vi "AllDataConcat.vi"(8 "error in (no error)":errorcluster, 11 "AllDataArray":T1[](array[typedef]) {"FlukeData"."DataAnalysisArray"."TimeStamp" format="%^<%.3X\n%x>T"; "FlukeData"."ModelDataArray"."FREQUENCY" format="%#_6f"; "FlukeData"."ModelDataArray"."TimeStamp" format="%^<%.3X\n%x>T"; "FlukeData"."PMUDataArray"."FREQUENCY" format="%#_6f"; "FlukeData"."PMUDataArray"."TimeStamp" format="%^<%.3X\n%x>T"; "NISTData"."DataAnlysisArray"."Time" format="%.6f"; "NISTData"."DataAnlysisArray"."TimeStamp" format="%^<%.3X\n%x>T"; "NISTData"."DUTDataArray"."TimeStamp" format="%^<%.3X\n%x>T"; "NISTData"."DUTDataArray"."Time" format="%.6f"; "NISTData"."NIDataArray"."TimeStamp" format="%^<%.3X\n%x>T"; "NISTData"."NIDataArray"."Time" format="%.6f"}) -> (0 "error out":errorcluster, 3 "AllData":T1 {"FlukeData"."DataAnalysisArray"."TimeStamp" format="%^<%.3X\n%x>T"; "FlukeData"."ModelDataArray"."FREQUENCY" format="%#_6f"; "FlukeData"."ModelDataArray"."TimeStamp" format="%^<%.3X\n%x>T"; "FlukeData"."PMUDataArray"."FREQUENCY" format="%#_6f"; "FlukeData"."PMUDataArray"."TimeStamp" format="%^<%.3X\n%x>T"; "NISTData"."DataAnlysisArray"."Time" format="%.6f"; "NISTData"."DataAnlysisArray"."TimeStamp" format="%^<%.3X\n%x>T"; "NISTData"."DUTDataArray"."TimeStamp" format="%^<%.3X\n%x>T"; "NISTData"."DUTDataArray"."Time" format="%.6f"; "NISTData"."NIDataArray"."TimeStamp" format="%^<%.3X\n%x>T"; "NISTData"."NIDataArray"."Time" format="%.6f"})   [LabVIEW 2014]
uses:
  typedefs/Alldata.ctl
  typedefs/NISTData.ctl
  typedefs/NIDataArray.ctl
  typedefs/NIData.ctl
  typedefs/PhasorRectangular.ctl
  typedefs/DUTData.ctl
  typedefs/NICalcAnalysis.ctl
  typedefs/CalcPhasorError.ctl
  typedefs/PlotDataArrays.ctl
  typedefs/PmuRawDataCluster.ctl
  typedefs/CalcAnalysis.ctl
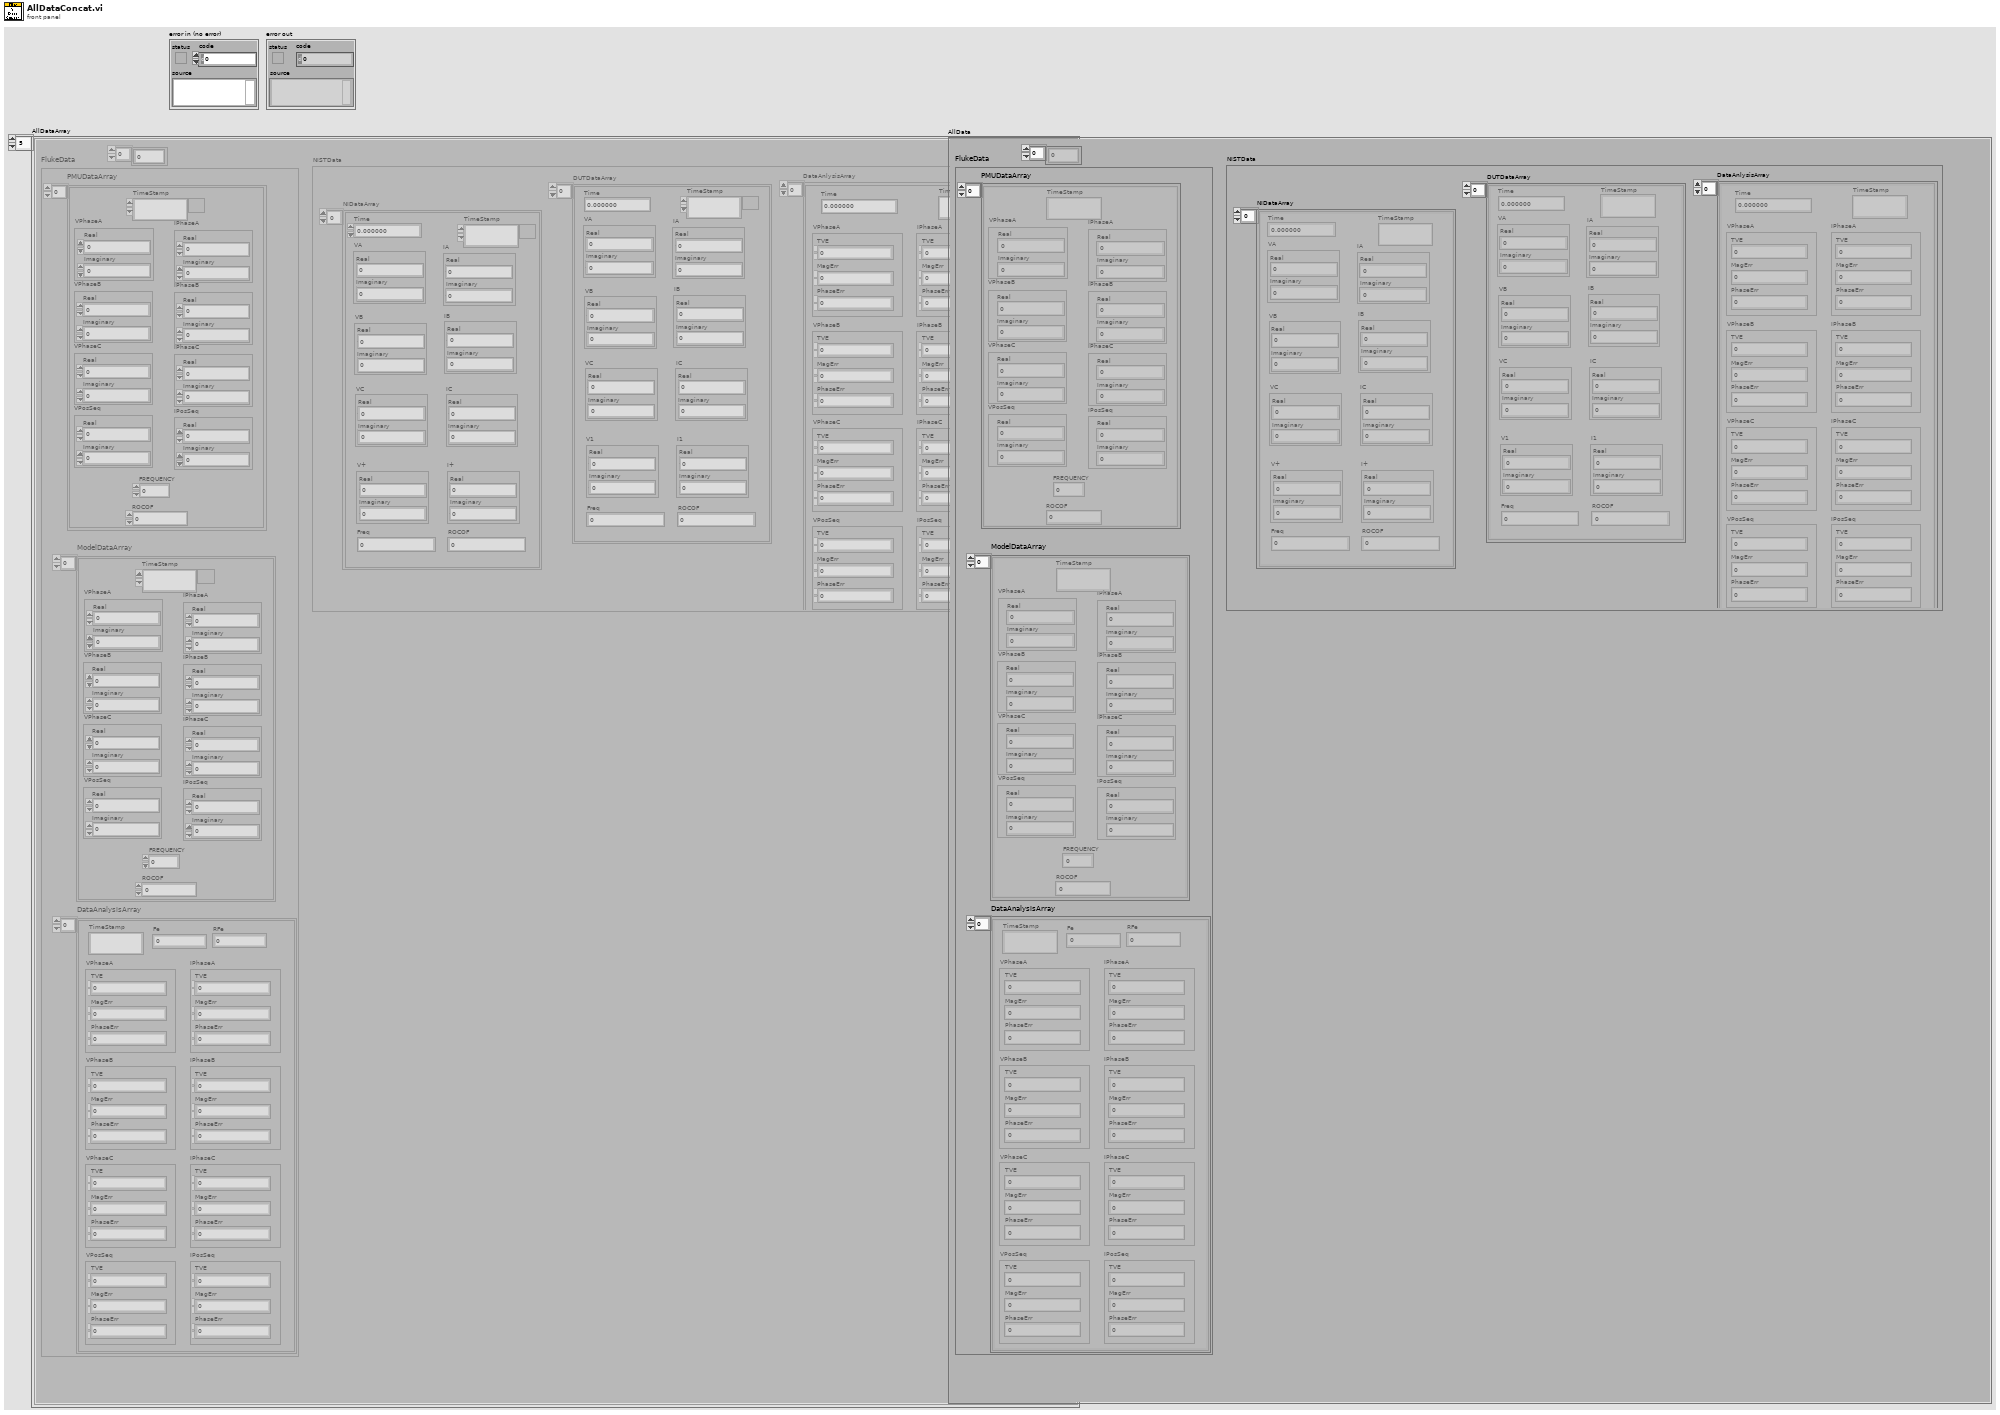
[diagram p1: front panel]
types:
  T1 = typedef "Alldata.ctl" = cluster{"NISTData":T2, "FlukeData":T9, "Params":dbl[]}
  T2 = typedef "NISTData.ctl" = cluster{"NIDataArray":T3, "DUTDataArray":T6[], "DataAnlysisArray":T7[]}
  T3 = typedef "NIDataArray.ctl" = T4[]
  T4 = typedef "NIData.ctl" = cluster{"Time":dbl, "VA":T5, "VB":T5, "VC":T5, "V+":T5, "IA":T5, "IB":T5, "IC":T5, "I+":T5, "Freq":dbl, "ROCOF":dbl, "TimeStamp":timestamp}
  T5 = typedef "PhasorRectangular.ctl" = cluster{"Real":dbl, "Imaginary":dbl}
  T6 = typedef "DUTData.ctl" = cluster{"Time":dbl, "VA":T5, "VB":T5, "VC":T5, "V1":T5, "IA":T5, "IB":T5, "IC":T5, "I1":T5, "Freq":dbl, "ROCOF":dbl, "TimeStamp":timestamp}
  T7 = typedef "NICalcAnalysis.ctl" = cluster{"Time":dbl, "VPhaseA":T8, "VPhaseB":T8, "VPhaseC":T8, "VPosSeq":T8, "IPhaseA":T8, "IPhaseB":T8, "IPhaseC":T8, "IPosSeq":T8, "Fe":dbl, "RFe":dbl, "TimeStamp":timestamp}
  T8 = typedef "CalcPhasorError.ctl" = cluster{"TVE":dbl, "MagErr":dbl, "PhaseErr":dbl}
  T9 = typedef "PlotDataArrays.ctl" = cluster{"PMUDataArray":T10[], "ModelDataArray":T10[], "DataAnalysisArray":T11[]}
  T10 = typedef "PmuRawDataCluster.ctl" = cluster{"TimeStamp":timestamp, "VPhaseA":T5, "VPhaseB":T5, "VPhaseC":T5, "VPosSeq":T5, "IPhaseA":T5, "IPhaseB":T5, "IPhaseC":T5, "IPosSeq":T5, "FREQUENCY":dbl, "ROCOF":sgl}
  T11 = typedef "CalcAnalysis.ctl" = cluster{"TimeStamp":timestamp, "VPhaseA":T8, "VPhaseB":T8, "VPhaseC":T8, "VPosSeq":T8, "IPhaseA":T8, "IPhaseB":T8, "IPhaseC":T8, "IPosSeq":T8, "Fe":dbl, "RFe":dbl}
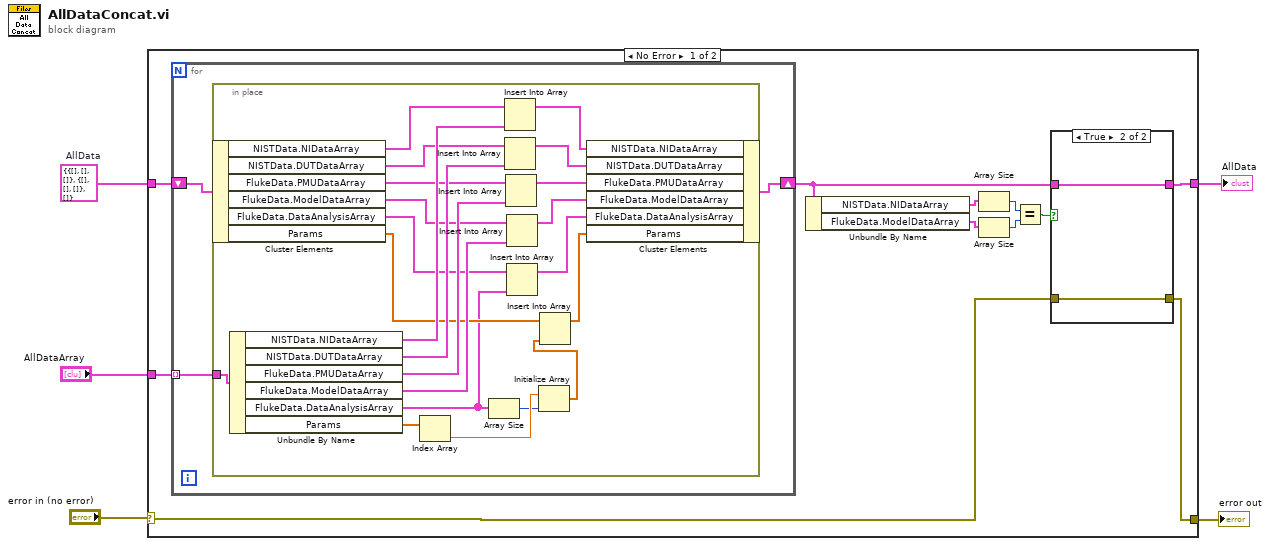
[diagram p0: block diagram]
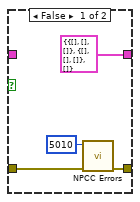
[diagram p2: hidden frame]
diagram:
  w5 = T1 {"NISTData"={"NIDataArray"=[], "DUTDataArray"=[], "DataAnlysisArray"=[]}, "FlukeData"={"PMUDataArray"=[], "ModelDataArray"=[], "DataAnalysisArray"=[]}, "Params"=[]}  # AllData
  n1 = case shown="No Error" "error in (no error)" {
    selector: "error in (no error)" -> [w7 w48]
    tunnel: w5 -> [w16 w49]
    tunnel: "AllDataArray" -> [w15 _]
    tunnel: [w9 w49] -> w3
    tunnel: [w6 w48] -> w1
    frame No Error {
      n2 = for {
        tunnel: w15 -> [w23] mode=indexing
        shift-right: [w24] -> w8
        shift-left: w16 -> [w25]
        n3 = in-place {
          in-place-border: w23 -> [w42]
          n4 = in-place-cluster #1(w25) -> ("NISTData.NIDataArray"=w40:T3, "NISTData.DUTDataArray"=w39:T6[], "FlukeData.PMUDataArray"=w37:T10[], "FlukeData.ModelDataArray"=w35:T10[], "FlukeData.DataAnalysisArray"=w33:T11[], "Params"=w31:dbl[])
          n5 = Unbundle By Name(w42) -> ("NISTData.NIDataArray"=w41:T3, "NISTData.DUTDataArray"=w38:T6[], "FlukeData.PMUDataArray"=w36:T10[], "FlukeData.ModelDataArray"=w34:T10[], "FlukeData.DataAnalysisArray"=w29:T11[], "Params"=w32:dbl[])
          n6 = Index Array(array=w32) -> (element=w28:dbl)  [unwired: 1 in]
          n7 = Array Size(array=w29) -> (size(s)=w27:i32)
          n8 = Insert Into Array(array=w40, new element=w41) -> (w47:T3)  [unwired: 1 in]
          n9 = Insert Into Array(array=w39, new element=w38) -> (w46:T6[])  [unwired: 1 in]
          n10 = Insert Into Array(array=w37, new element=w36) -> (w45:T10[])  [unwired: 1 in]
          n11 = Insert Into Array(array=w35, new element=w34) -> (w44:T10[])  [unwired: 1 in]
          n12 = Insert Into Array(array=w33, new element=w29) -> (w43:T11[])  [unwired: 1 in]
          n13 = Initialize Array(w28, w27) -> (w26:dbl[])
          n14 = Insert Into Array(array=w31, new element=w26) -> (w30:dbl[])  [unwired: 1 in]
          n15 = in-place-cluster #1("NISTData.NIDataArray"=w47, "NISTData.DUTDataArray"=w46, "FlukeData.PMUDataArray"=w45, "FlukeData.ModelDataArray"=w44, "FlukeData.DataAnalysisArray"=w43, "Params"=w30) -> (w24:T1)
        }
      }
      n16 = Unbundle By Name(w8) -> ("NISTData.NIDataArray"=w11:T3, "FlukeData.ModelDataArray"=w12:T10[])
      n17 = Array Size(array=w11) -> (size(s)=w14:i32)
      n18 = Array Size(array=w12) -> (size(s)=w13:i32)
      n19 = Equal?(x=w14, y=w13) -> (x = y?=w10:bool)
      n20 = case shown="True" w10 {
        tunnel: [T1 {"NISTData"={"NIDataArray"=[], "DUTDataArray"=[], "DataAnlysisArray"=[]}, "FlukeData"={"PMUDataArray"=[], "ModelDataArray"=[], "DataAnalysisArray"=[]}, "Params"=[]} ("AllData") w22] -> w9
        tunnel: w8 -> [_ w22]
        tunnel: [w18 w21] -> w6
        tunnel: w7 -> [w19 w21]
        frame False {
          n21 = call "NPCC Errors.vi"("error in (no error)"=w19, "[error code] (0)"=5010 ("error code (no error:0)")) -> ("error out"=w18:errorcluster)  [unwired: 9 in]
        }
        frame True {
        }
      }
    }
    frame Error {
    }
  }
  "AllData" <- w3
  "error out" <- w1
